vi "XML to Name Value.vi"(0 "XML In":string, 11 "Error In":errorcluster) -> (4 "Name Value CSV":string, 8 "Name Value Array":string[][](array[string]), 15 "Error Out":errorcluster)   [LabVIEW 2020]
uses:
  <vilib>/regexp/Match Regular Expression.xnode
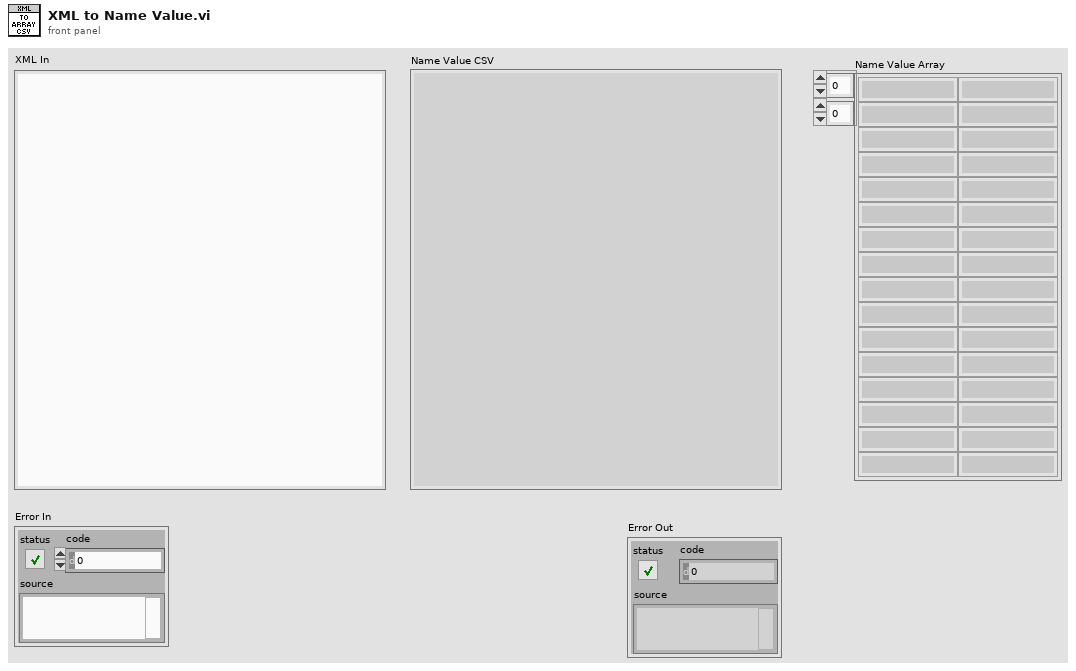
[diagram p1: front panel]
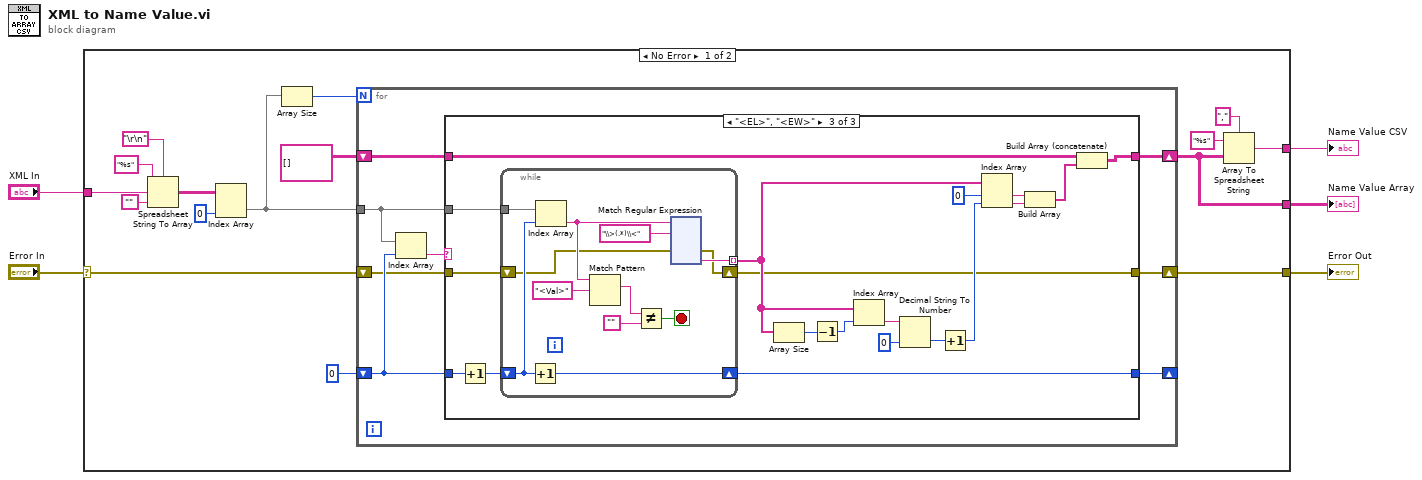
[diagram p0: block diagram]
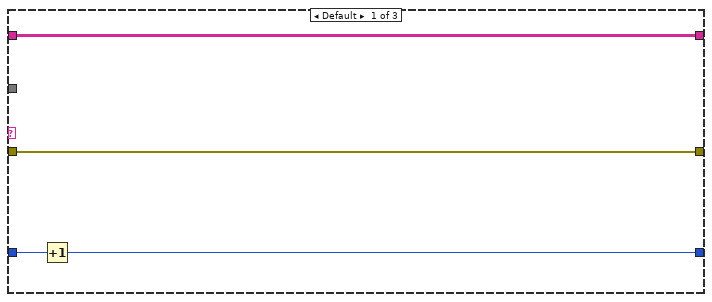
[diagram p2: hidden frame]
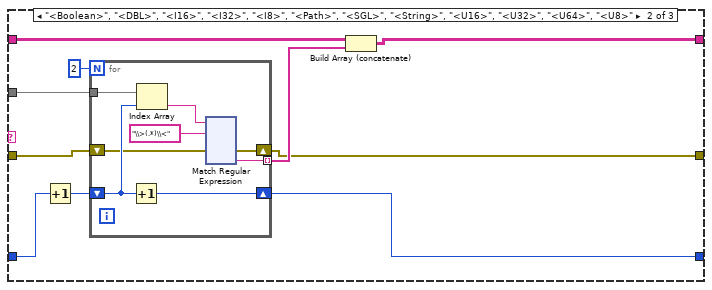
[diagram p3: hidden frame]
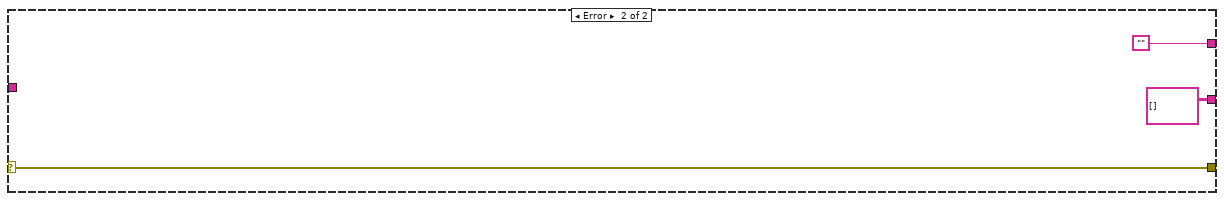
[diagram p4: hidden frame]
diagram:
  n1 = case shown="No Error" "Error In" {
    selector: "Error In" -> [w8 w316]
    tunnel: [w10 ""] -> w5
    tunnel: "XML In" -> [w9 _]
    tunnel: [w7 w316] -> w2
    tunnel: [w6 string[][] []] -> w1
    frame No Error {
      n2 = Spreadsheet String To Array(delimiter (Tab)="\r\n", format string="%s", spreadsheet string=w9, array type (2D Dbl)="") -> (array=w18:string[][])
      n3 = Index Array(array=w18, index (col)=0 ("disabled index (col)")) -> (element=w14:string[])  [unwired: 1 in]
      n4 = Array Size(array=w14) -> (size(s)=w13:i32)
      n5 = for {
        N: w13 -> [_]
        tunnel: w14 -> [w26]
        shift-right: [w27] -> _
        shift-left: 0 -> [w28]
        shift-right: [w24] -> w6
        shift-left: string[][] [] -> [w25]
        shift-right: [w22] -> w7
        shift-left: w8 -> [w23]
        n6 = Index Array(array=w26, index=w28) -> (element=w29:string)
        n7 = case shown="\"<EL>\", \"<EW>\"" w29 {
          tunnel: w28 -> [w33 w43 w185]
          tunnel: [w32 w39 w181] -> w27
          tunnel: w26 -> [_ w42 w183]
          tunnel: w25 -> [w31 w38 w186]
          tunnel: [w31 w36 w184] -> w24
          tunnel: w23 -> [w30 w35 w169]
          tunnel: [w30 w34 w168] -> w22
          frame Default {
            n8 = Increment(x=w33) -> (x+1=w32:i32)
          }
          frame "<Boolean>", "<DBL>", "<I16>", "<I32>", "<I8>", "<Path>", "<SGL>", "<String>", "<U16>", "<U32>", "<U64>", "<U8>" {
            n9 = Increment(x=w43) -> (x+1=w41:i32)
            n10 = for {
              N: 2 -> [_]
              shift-right: [w49] -> w39
              shift-left: w41 -> [w50]
              tunnel: w42 -> [w51]
              tunnel: [w46] -> w37 mode=indexing
              shift-right: [w44] -> w34
              shift-left: w35 -> [w45]
              n11 = Increment(x=w50) -> (x+1=w49:i32)
              n12 = Index Array(array=w51, index=w50) -> (element=w47:string)
              n13 = xnode "Match Regular Expression"("input string"=w47, "regular expression"="\\>(.*)\\<", "error in"=w45) -> ("error out"=w44:errorcluster, "submatch 1"=w46:string)  [unwired: 3 in, 4 out]
            }
            n14 = Build Array (concatenate)(w38, w37) -> (w36:string[][])
          }
          frame "<EL>", "<EW>" {
            n15 = Increment(x=w185) -> (x+1=w182:i32)
            n16 = while {
              tunnel: w183 -> [w198]
              shift-right: [w196] -> w181
              shift-left: w182 -> [w197]
              tunnel: [w194] -> w175 mode=indexing
              shift-right: [w187] -> w168
              shift-left: w169 -> [w188]
              stop <- w189 stop-if-true
              n17 = Increment(x=w197) -> (x+1=w196:i32)
              n18 = Index Array(array=w198, index=w197) -> (element=w192:string)
              n19 = Match Pattern(string=w192, regular expression="<Val>") -> (match substring=w191:string)  [unwired: 1 in, 3 out]
              n20 = Not Equal?(x=w191, y="") -> (x != y?=w189:bool)
              n21 = xnode "Match Regular Expression"("input string"=w192, "regular expression"="\\>(.*)\\<", "error in"=w188) -> ("error out"=w187:errorcluster, "submatch 1"=w194:string)  [unwired: 3 in, 4 out]
            }
            n22 = Array Size(array=w175) -> (size(s)=w177:i32)
            n23 = Decrement(x=w177) -> (x-1=w174:i32)
            n24 = Index Array(array=w175, index=w174) -> (element=w173:string)
            n25 = Decimal String To Number(string=w173, default (0L)=0 ("default (0 I32)")) -> (number=w171:i32)  [unwired: 1 in, 1 out]
            n26 = Increment(x=w171) -> (x+1=w170:i32)
            n27 = Index Array(array=w175, index #1=0 ("index"), index #2=w170) -> (element #1=w178:string, element #2=w176:string)
            n28 = Build Array(w178, w176) -> (w180:string[])
            n29 = Build Array (concatenate)(w186, w180) -> (w184:string[][])
          }
        }
      }
      n30 = Array To Spreadsheet String(delimiter (Tab)=",", array=w6, 3:"%s" ("format string")) -> (spreadsheet string=w10:string)
    }
    frame Error {
    }
  }
  "Name Value CSV" <- w5
  "Error Out" <- w2
  "Name Value Array" <- w1
